vi "Ka2tesla.vi"(2 "Magnet Current [kA]":dbl=1.0 format="%.4f") -> (0 "Field":dbl=1.0 format="%.4f")   [LabVIEW 2020]
uses:
  PS Comm Globals.vi
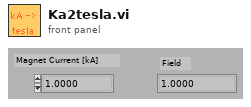
[diagram p1: front panel]
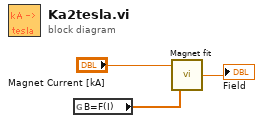
[diagram p0: block diagram]
diagram:
  n1 = global read "PS Comm Globals.vi" "B=F(I)"() -> (w2:dbl[])
  n2 = call "Magnet fit.vi"("Coefficients"=w2, "Magnet Parameter"="Magnet Current [kA]") -> ("Conjugate Parameter"=→"Field":dbl)
